vi "BioFLEX Board Switch TEENSY v2.vi"() -> ()   [LabVIEW 2015]
uses:
  <vilib>/Instr/_visa.llb/VISA Configure Serial Port (Instr).vi
panel:
  in  "MUX 4":T1(ring)
  in  "MUX 3":T1(ring)
  in  "MUX 2":T1(ring)
  in  "MUX 1":T1(ring)
  in  "MUX 4 Enable":bool=TRUE
  in  "MUX 3 Enable":bool=TRUE
  in  "MUX 1 Enable":bool=TRUE
  in  "MUX 2 Enable":bool=TRUE
  in  "stop":bool
  out "error out":errorcluster
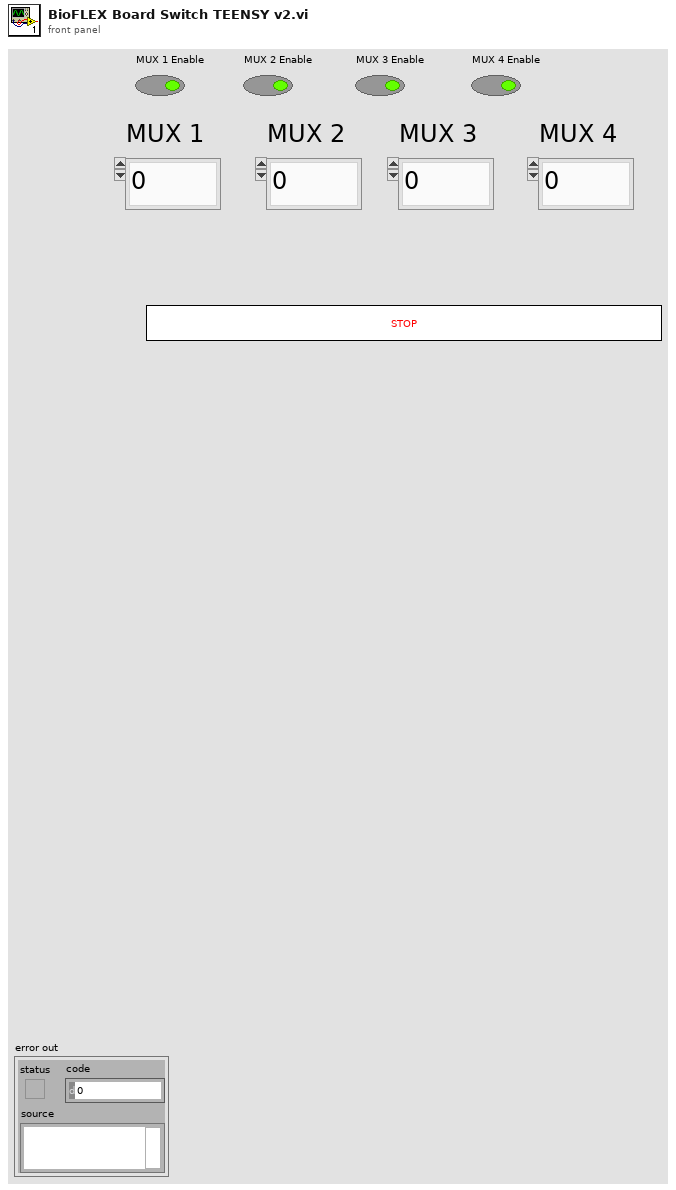
[diagram p1: front panel]
types:
  T1 = enum16{"0", "1", "2", "3", "4", "5", "6", "7", "8", "9", "10", "11", "12", "13", "14", "15", "16"}
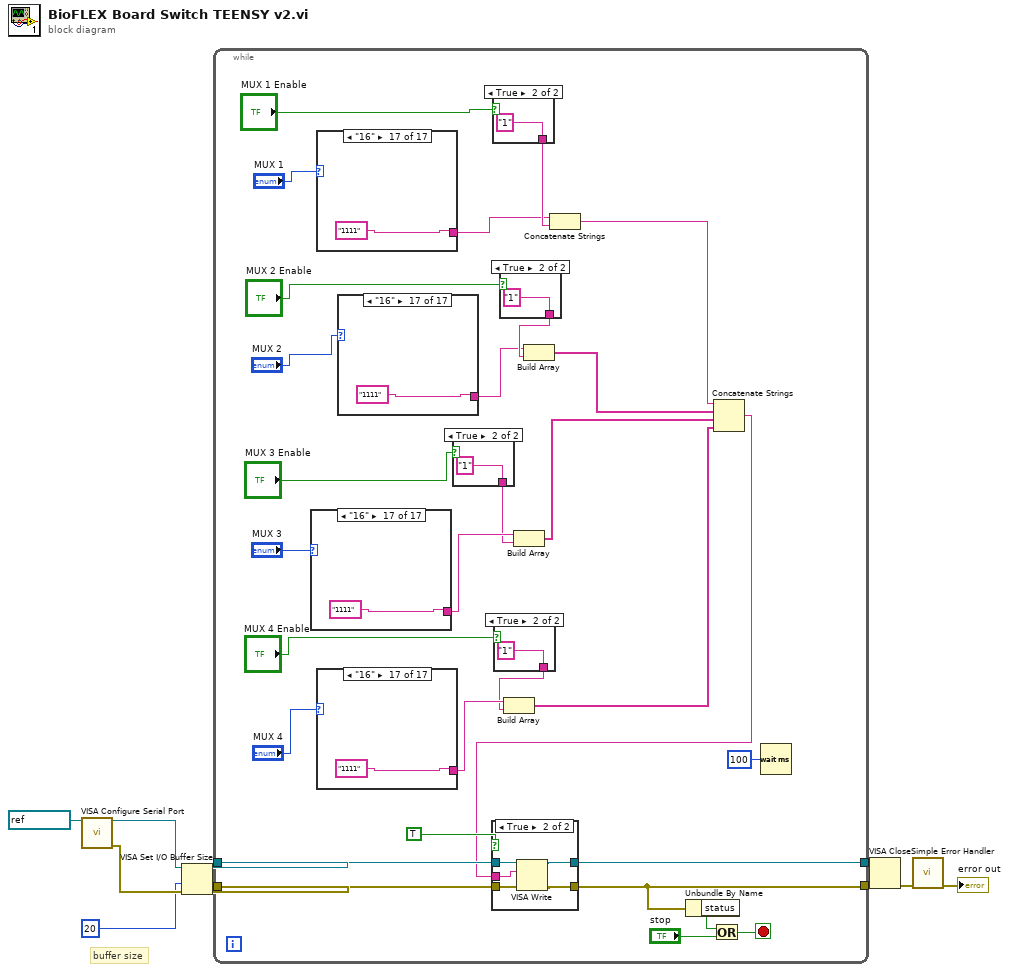
[diagram p0: block diagram]
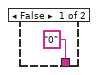
[diagram p2: hidden frame]
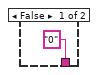
[diagram p3: hidden frame]
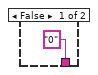
[diagram p4: hidden frame]
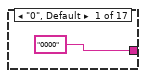
[diagram p5: hidden frame]
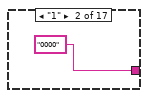
[diagram p6: hidden frame]
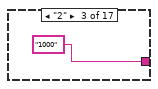
[diagram p7: hidden frame]
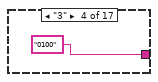
[diagram p8: hidden frame]
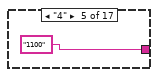
[diagram p9: hidden frame]
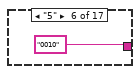
[diagram p10: hidden frame]
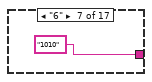
[diagram p11: hidden frame]
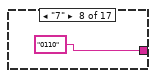
[diagram p12: hidden frame]
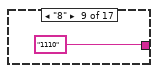
[diagram p13: hidden frame]
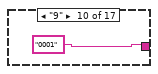
[diagram p14: hidden frame]
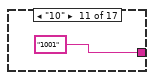
[diagram p15: hidden frame]
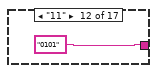
[diagram p16: hidden frame]
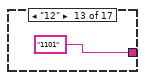
[diagram p17: hidden frame]
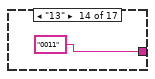
[diagram p18: hidden frame]
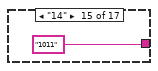
[diagram p19: hidden frame]
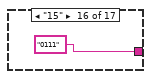
[diagram p20: hidden frame]
diagram:
  # "buffer size"
  n1 = call-poly "VISA Configure Serial Port"("VISA resource name"=refnum<visa-resource-name> "COM4") -> ("VISA resource name out"=w9:refnum<visa-resource-name>, "error out"=w10:errorcluster)  [unwired: 13 in]
  n2 = VISA Set I/O Buffer Size(VISA resource name=w9, size (4096)=u32 20 ("buffer size"), error in (no error)=w10) -> (VISA resource name out=w8:refnum<visa-resource-name>, error out=w7:errorcluster)  [unwired: 1 in]
  n3 = while {
    tunnel: w8 -> [w37]
    tunnel: w7 -> [w36]
    tunnel: [w33] -> w2
    tunnel: [w32] -> w3
    stop <- w38 stop-if-true
    n4 = case shown="\"16\"" "MUX 3" {
      tunnel: ["0000" "0000" "1000" "0100" "1100" "0010" "1010" "0110" "1110" "0001" "1001" "0101" "1101" "0011" "1011" "0111" "1111"] -> w24
      frame "0", Default {
      }
      frame "1" {
      }
      frame "2" {
      }
      frame "3" {
      }
      frame "4" {
      }
      frame "5" {
      }
      frame "6" {
      }
      frame "7" {
      }
      frame "8" {
      }
      frame "9" {
      }
      frame "10" {
      }
      frame "11" {
      }
      frame "12" {
      }
      frame "13" {
      }
      frame "14" {
      }
      frame "15" {
      }
      frame "16" {
      }
    }
    n5 = case shown="\"16\"" "MUX 1" {
      tunnel: ["0000" "0000" "1000" "0100" "1100" "0010" "1010" "0110" "1110" "0001" "1001" "0101" "1101" "0011" "1011" "0111" "1111"] -> w28
      frame "0", Default {
      }
      frame "1" {
      }
      frame "2" {
      }
      frame "3" {
      }
      frame "4" {
      }
      frame "5" {
      }
      frame "6" {
      }
      frame "7" {
      }
      frame "8" {
      }
      frame "9" {
      }
      frame "10" {
      }
      frame "11" {
      }
      frame "12" {
      }
      frame "13" {
      }
      frame "14" {
      }
      frame "15" {
      }
      frame "16" {
      }
    }
    n6 = case shown="\"16\"" "MUX 4" {
      tunnel: ["0000" "0000" "1000" "0100" "1100" "0010" "1010" "0110" "1110" "0001" "1001" "0101" "1101" "0011" "1011" "0111" "1111"] -> w23
      frame "0", Default {
      }
      frame "1" {
      }
      frame "2" {
      }
      frame "3" {
      }
      frame "4" {
      }
      frame "5" {
      }
      frame "6" {
      }
      frame "7" {
      }
      frame "8" {
      }
      frame "9" {
      }
      frame "10" {
      }
      frame "11" {
      }
      frame "12" {
      }
      frame "13" {
      }
      frame "14" {
      }
      frame "15" {
      }
      frame "16" {
      }
    }
    n7 = case shown="\"16\"" "MUX 2" {
      tunnel: ["0000" "0000" "1000" "0100" "1100" "0010" "1010" "0110" "1110" "0001" "1001" "0101" "1101" "0011" "1011" "0111" "1111"] -> w17
      frame "0", Default {
      }
      frame "1" {
      }
      frame "2" {
      }
      frame "3" {
      }
      frame "4" {
      }
      frame "5" {
      }
      frame "6" {
      }
      frame "7" {
      }
      frame "8" {
      }
      frame "9" {
      }
      frame "10" {
      }
      frame "11" {
      }
      frame "12" {
      }
      frame "13" {
      }
      frame "14" {
      }
      frame "15" {
      }
      frame "16" {
      }
    }
    n8 = case shown="True" "MUX 3 Enable" {
      tunnel: ["0" "1"] -> w15
      frame False {
      }
      frame True {
      }
    }
    n9 = case shown="True" "MUX 1 Enable" {
      tunnel: ["0" "1"] -> w29
      frame False {
      }
      frame True {
      }
    }
    n10 = case shown="True" "MUX 4 Enable" {
      tunnel: ["0" "1"] -> w13
      frame False {
      }
      frame True {
      }
    }
    n11 = case shown="True" "MUX 2 Enable" {
      tunnel: ["0" "1"] -> w18
      frame False {
      }
      frame True {
      }
    }
    n12 = Build Array(w23, w13) -> (w11:string[])
    n13 = Build Array(w24, w15) -> (w14:string[])
    n14 = Build Array(w17, w18) -> (w16:string[])
    n15 = Concatenate Strings(w28, w29) -> (w12:string)
    n16 = Concatenate Strings(w12, w16, w14, w11) -> (w27:string)
    n17 = case shown="True" TRUE ("write") {
      tunnel: w37 -> [w118 w123]
      tunnel: w36 -> [w117 w122]
      tunnel: [w118 w121] -> w33
      tunnel: [w117 w120] -> w32
      tunnel: w27 -> [_ w119]
      frame False {
      }
      frame True {
        n18 = VISA Write(VISA resource name=w123, write buffer=w119, error in (no error)=w122) -> (VISA resource name out=w121:refnum<visa-resource-name>, error out=w120:errorcluster)  [unwired: 1 out]
      }
    }
    n19 = Unbundle By Name(w32) -> ("status"=w40:bool)
    n20 = Or(x=w40, y="stop") -> (x .or. y?=w38:bool)
    n21 = Wait (ms)(milliseconds to wait=u32 100) -> ()  [unwired: 1 out]
  }
  n22 = VISA Close(VISA resource name=w2, error in (no error)=w3) -> (error out=w4:errorcluster)
  n23 = call <vilib>:"Simple Error Handler.vi"("error in (no error)"=w4) -> ("error out"=→"error out":errorcluster)  [unwired: 4 in, 4 out]
